vi "LoadArmPressureAndCalcIndex.vi"(8 "error in (no error)":errorcluster, 11 "Path":path) -> (0 "error out":errorcluster, 2 "Armpressure":dbl, 3 "Path Out":path)   [LabVIEW 2013, in "main.lvlib"]
uses:
  main.lvlib
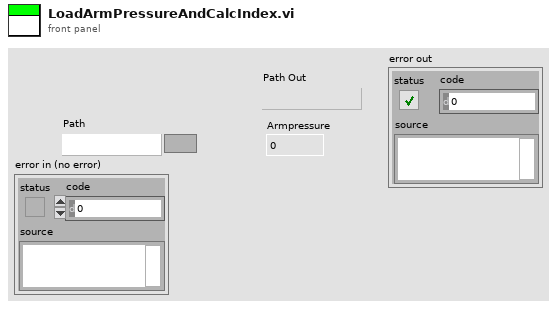
[diagram p1: front panel]
types:
  T1 = cluster{"sys":dbl, "dia":dbl, "puls":dbl, "date":string, "time":string, "code":string, "serial":string, "temp":dbl, "activity":string}[]
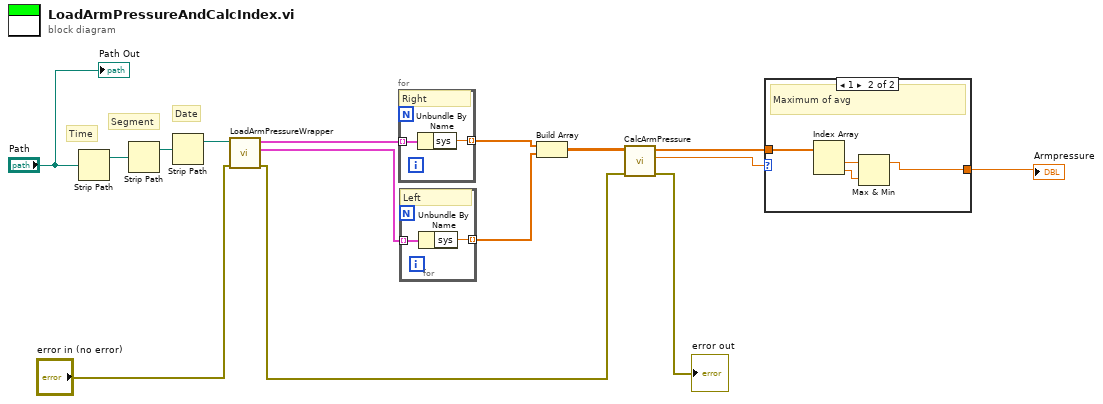
[diagram p0: block diagram]
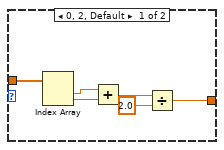
[diagram p2: hidden frame]
diagram:
  # "Date"
  # "Segment"
  # "Time"
  n1 = Strip Path(path="Path") -> (stripped path=w14:path)  [unwired: 1 out]
  n2 = Strip Path(path=w14) -> (stripped path=w13:path)  [unwired: 1 out]
  n3 = Strip Path(path=w13) -> (stripped path=w6:path)  [unwired: 1 out]
  n4 = call "LoadArmPressureWrapper.vi"("error in"="error in (no error)", "File dir"=w6) -> ("error out"=w1:errorcluster, "Armpressure Left"=w7:T1, "Armpressure Right"=w8:T1)  [unwired: 7 in]
  n5 = for {
    tunnel: w8 -> [w17] mode=indexing
    tunnel: [w16] -> w5 mode=indexing
    # "Right"
    n6 = Unbundle By Name(w17) -> ("sys"=w16:dbl)
  }
  n7 = for {
    tunnel: w7 -> [w19] mode=indexing
    tunnel: [w18] -> w4 mode=indexing
    # "Left"
    n8 = Unbundle By Name(w19) -> ("sys"=w18:dbl)
  }
  n9 = Build Array(w5, w4) -> (w3:dbl[][])
  n10 = call "CalcArmPressure.vi"("error in (no error)"=w1, "Armpres"=w3) -> ("error out"=→"error out":errorcluster, "Method"=w10:dbl, "Array Out"=w12:dbl[])  [unwired: 7 in]
  n11 = case shown="1" w10 {
    tunnel: w12 -> [w25 w29]
    tunnel: [w22 w26] -> w9
    frame 0, 2, Default {
      n12 = Index Array(array=w25) -> (element #1=w21:dbl, element #2=w20:dbl)  [unwired: 2 in]
      n13 = Add(x=w21, y=w20) -> (x+y=w23:dbl)
      n14 = Divide(x=w23, y=2.0) -> (x/y=w22:dbl)
    }
    frame 1 {
      # "Maximum of avg"
      n15 = Index Array(array=w29) -> (element #1=w28:dbl, element #2=w27:dbl)  [unwired: 2 in]
      n16 = Max & Min(x=w28, y=w27) -> (max(x,y)=w26:dbl)  [unwired: 1 out]
    }
  }
  "Armpressure" <- w9
  "Path Out" <- "Path"
